vi "CRYPEAQ CBMapping.vi"(8 "Version":u16(ring) items=["Basic", "Advance", "My"], 10 "Fs":dbl=48000.0, 11 "NF":dbl=2048.0) -> (0 "Uu":dbl[](array[numeric]), 1 "ku":i32[](array[numeric]), 2 "Ul":dbl[](array[numeric]), 3 "kl":i32[](array[numeric]), 4 "fc":dbl[](array[numeric]), 5 "fu":dbl[](array[numeric]), 6 "Nc":i32, 7 "fl":dbl[](array[numeric]))   [LabVIEW 2013]
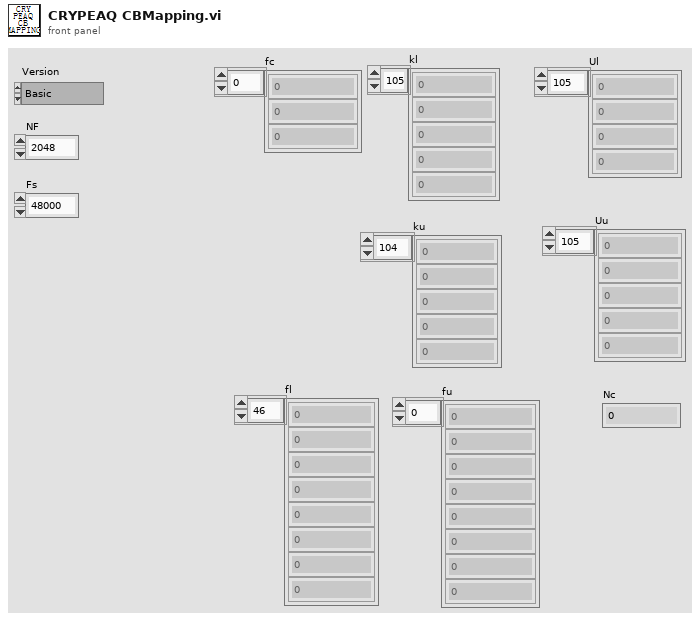
[diagram p1: front panel]
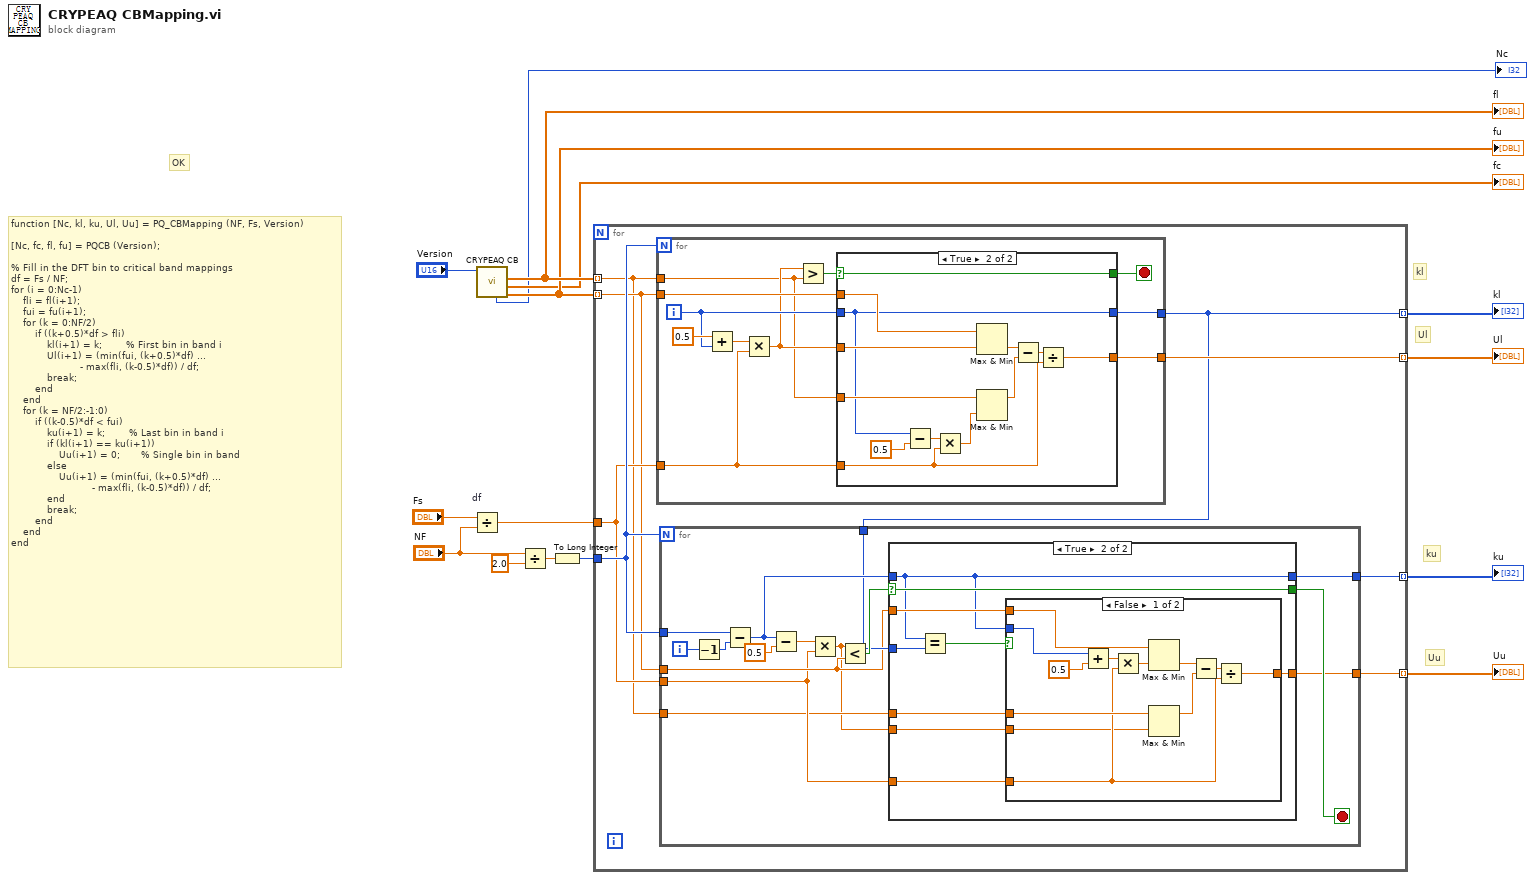
[diagram p0: block diagram]
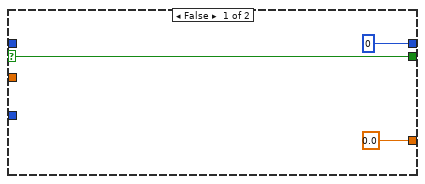
[diagram p2: hidden frame]
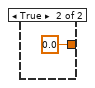
[diagram p3: hidden frame]
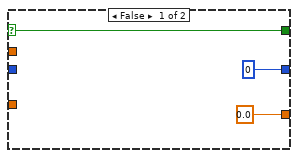
[diagram p4: hidden frame]
diagram:
  # "OK"
  # "function [Nc, kl, ku, Ul, Uu] = PQ_CBMapping (NF, Fs, Version)\n\n[Nc, fc, fl, fu] = PQCB (Version);\n\n% Fill in the DFT bin to critical band mappings\ndf = Fs / NF;\nfor (i = 0:Nc-1)\n    fli = fl(i+1);\n    fui = fu(i+1);\n    for (k = 0:NF/2)\n        if ((k+0.5)*df > fli)\n            kl(i+1) = k;        % First bin in band i\n            Ul(i+1) = (min(fui, (k+0.5)*df) ...\n                       - max(fli, (k-0.5)*df)) / df;\n            break;\n        end\n    end\n    for (k = NF/2:-1:0)\n        if ((k-0.5)*df < fui)\n            ku(i+1) = k;        % Last bin in band i\n            if (kl(i+1) == ku(i+1))\n                Uu(i+1) = 0;       % Single bin in band\n            else\n                Uu(i+1) = (min(fui, (k+0.5)*df) ...\n                           - max(fli, (k-0.5)*df)) / df;\n            end\n            break;\n        end\n    end\nend"
  # "Uu"
  # "ku"
  # "Ul"
  # "kl"
  n1 = Divide "df"(x="Fs", y="NF") -> (x/y=w8:dbl)
  n2 = call "CRYPEAQ CB.vi"("Version"="Version") -> ("fu"=w13:dbl[], "fc"=→"fc":dbl[], "fl"=w14:dbl[], "Nc"=→"Nc":i32)  [unwired: 6 in, 1 out]
  "fu" <- w13
  "fl" <- w14
  n3 = Divide(x="NF", y=2.0) -> (x/y=w10:dbl)
  n4 = To Long Integer(number=w10) -> (32bit integer=w9:i32)
  n5 = for {
    tunnel: w14 -> [w16] mode=indexing
    tunnel: w13 -> [w20] mode=indexing
    tunnel: w9 -> [w23]
    tunnel: w8 -> [w21]
    tunnel: [w18] -> w6 mode=indexing
    tunnel: [w22] -> w5 mode=indexing
    tunnel: [w19] -> w7 mode=indexing
    tunnel: [w17] -> w4 mode=indexing
    n6 = for {
      N: w23 -> [_]
      tunnel: w16 -> [w66]
      tunnel: w20 -> [w68]
      tunnel: w21 -> [w65]
      tunnel: [w69] -> w18
      tunnel: [w64] -> w22
      i -> [w70]
      stop <- w71 stop-if-true
      n7 = Add(x=0.5, y=w70) -> (x+y=w73:dbl)
      n8 = Multiply(x=w73, y=w65) -> (x*y=w67:dbl)
      n9 = Greater?(x=w67, y=w66) -> (0:w72:bool)
      n10 = case shown="True" w72 {
        selector: w72 -> [w77 w90]
        tunnel: [w77 w90] -> w71
        tunnel: w70 -> [_ w85]
        tunnel: [0 w85] -> w69
        tunnel: w68 -> [_ w89]
        tunnel: w67 -> [_ w88]
        tunnel: w66 -> [_ w87]
        tunnel: w65 -> [_ w79]
        tunnel: [0.0 w78] -> w64
        frame False {
        }
        frame True {
          n11 = Subtract(x=w85, y=0.5) -> (x-y=w86:dbl)
          n12 = Multiply(x=w86, y=w79) -> (x*y=w83:dbl)
          n13 = Max & Min(x=w89, y=w88) -> (min(x,y)=w82:dbl)  [unwired: 1 out]
          n14 = Max & Min(x=w87, y=w83) -> (max(x,y)=w81:dbl)  [unwired: 1 out]
          n15 = Subtract(x=w82, y=w81) -> (x-y=w80:dbl)
          n16 = Divide(x=w80, y=w79) -> (x/y=w78:dbl)
        }
      }
    }
    n17 = for {
      N: w23 -> [_]
      tunnel: w23 -> [w37]
      tunnel: w21 -> [w26]
      tunnel: w20 -> [w27]
      tunnel: [w30] -> w19
      tunnel: w18 -> [w29]
      tunnel: [w28] -> w17
      tunnel: w16 -> [w25]
      i -> [w38]
      stop <- w32 stop-if-true
      n18 = Decrement(x=w38) -> (x-1=w36:i32)
      n19 = Subtract(x=w37, y=w36) -> (x-y=w31:i32)
      n20 = Subtract(x=w31, y=0.5) -> (x-y=w34:dbl)
      n21 = Multiply(x=w34, y=w26) -> (x*y=w24:dbl)
      n22 = Less?(x=w24, y=w27) -> (x < y?=w33:bool)
      n23 = case shown="True" w33 {
        selector: w33 -> [w41 w50]
        tunnel: [w41 w50] -> w32
        tunnel: w27 -> [_ w49]
        tunnel: w25 -> [_ w48]
        tunnel: w26 -> [_ w47]
        tunnel: [0.0 w46] -> w28
        tunnel: w31 -> [_ w43]
        tunnel: [0 w43] -> w30
        tunnel: w29 -> [_ w45]
        tunnel: w24 -> [_ w42]
        frame False {
        }
        frame True {
          n24 = Equal?(x=w43, y=w45) -> (x = y?=w44:bool)
          n25 = case shown="False" w44 {
            tunnel: w49 -> [w62 _]
            tunnel: w48 -> [w61 _]
            tunnel: w43 -> [w59 _]
            tunnel: w47 -> [w54 _]
            tunnel: [w51 0.0] -> w46
            tunnel: w42 -> [w52 _]
            frame False {
              n26 = Add(x=w59, y=0.5) -> (x+y=w60:dbl)
              n27 = Multiply(x=w60, y=w54) -> (x*y=w53:dbl)
              n28 = Max & Min(x=w62, y=w53) -> (min(x,y)=w57:dbl)  [unwired: 1 out]
              n29 = Max & Min(x=w61, y=w52) -> (max(x,y)=w56:dbl)  [unwired: 1 out]
              n30 = Subtract(x=w57, y=w56) -> (x-y=w55:dbl)
              n31 = Divide(x=w55, y=w54) -> (x/y=w51:dbl)
            }
            frame True {
            }
          }
        }
      }
    }
  }
  "kl" <- w6
  "Ul" <- w5
  "ku" <- w7
  "Uu" <- w4
